vi "CloseInstrumentSession.vi"(8 "error in (no error)":errorcluster, 11 "NISTNiPxi6123 in":refnum<class "NiPxi6123.lvclass">) -> (0 "error out":errorcluster, 3 "NISTNiPxi6123 out":refnum<class "NiPxi6123.lvclass">)   [LabVIEW 2014, in "SamplerPlugins.lvlib" / "NiPxi6123.lvclass"]
uses:
  NiPxi6123.lvclass
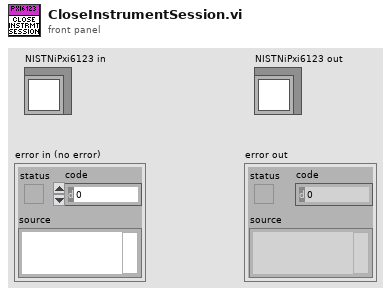
[diagram p1: front panel]
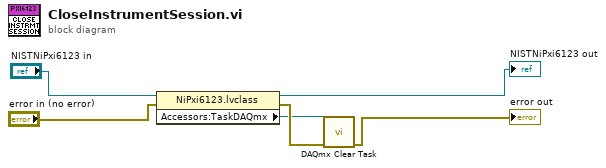
[diagram p0: block diagram]
diagram:
  n1 = property class="NiPxi6123.lvclass"(reference="NISTNiPxi6123 in", error in="error in (no error)") -> (reference out=→"NISTNiPxi6123 out":refnum<class "NiPxi6123.lvclass">, error out=w4:errorcluster, "Accessors:TaskDAQmx"=w3:refnum<k21>)
  n2 = call <vilib>:"DAQmx Clear Task.vi"("task in"=w3, "error in"=w4) -> ("error out"=→"error out":errorcluster)  [unwired: 13 in]
